vi "GetDataVersion.vi"(0 "session In":refnum<k35>, 5 "GEA2 Reference In":refnum<k24>, 11 "error In":errorcluster) -> (4 "session out":refnum<k35>, 8 "Data Version Out":cluster{"ERD Number":u16, "Data":string}[](array[cluster]), 15 "error out":errorcluster)   [LabVIEW 2023]
uses:
  D:/Common/LabVIEW GEA2 Toolkit/source/GEA3 DLL Source/GeaCommunication.dll
  Common/LabVIEW GEA2 Toolkit/source/GEA3 DLL Source/GeaCommunication.dll
  Common/LabVIEW GEA2 Toolkit/GEA3/type defs/Data Type.ctl
  Common/LabVIEW GEA2 Toolkit/GEA3/library/GEA2_Toolkit.lvlib
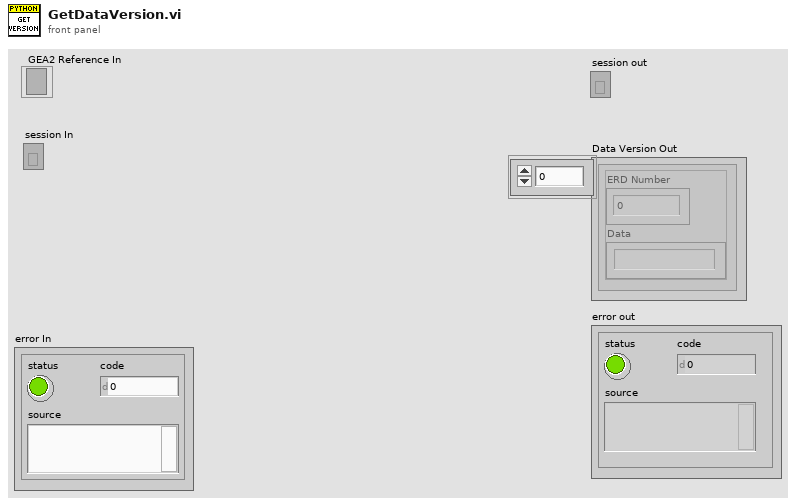
[diagram p1: front panel]
types:
  T1 = typedef "Data Type.ctl" = enum16{"string", "boolean", "uint8_t", "uint16_t", "uint32_t", "uint64_t", "int8_t", "int16_t", "int32_t", "int64_t"}
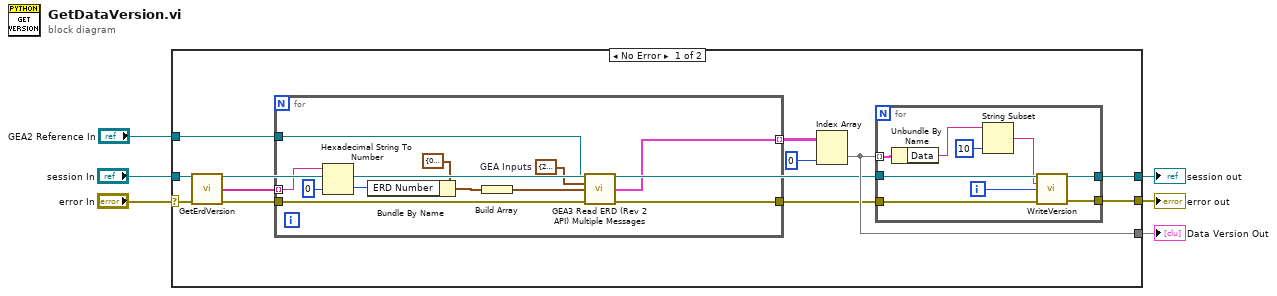
[diagram p0: block diagram]
diagram:
  n1 = case shown="No Error" "error In" {
    selector: "error In" -> [w8 w40]
    tunnel: [w15 _] -> w1
    tunnel: "GEA2 Reference In" -> [w11 _]
    tunnel: "session In" -> [w10 w39]
    tunnel: [w9 w39] -> w3
    tunnel: [w7 w40] -> w2
    frame No Error {
      n2 = call "GetErdVersion.vi"("session in"=w10, "error In"=w8) -> ("session Out"=w14:refnum<k35>, "Erds To Read"=w18:string[], "error Out"=w13:errorcluster)  [unwired: 11 in]
      n3 = for {
        tunnel: w11 -> [w38]
        tunnel: w13 -> [w37]
        tunnel: w18 -> [w32] mode=indexing
        tunnel: [w30] -> w17 mode=indexing
        tunnel: [w29] -> w12
        w36 = cluster{"Source":u8, "Destination":u8} {"Source"=229, "Destination"=192}  # GEA Inputs
        n4 = Hexadecimal String To Number(string=w32, default (0uL)=u16 0 ("ERD Number")) -> (number=w31:u16)  [unwired: 1 in, 1 out]
        n5 = Bundle By Name(cluster=cluster{"ERD Number":u16, "Data Type":T1} {"ERD Number"=0, "Data Type"=enum."string"} ("ERD Read Data In"), "ERD Number"=w31) -> (w35:cluster{"ERD Number":u16, "Data Type":T1})
        n6 = Build Array(w35) -> (w33:cluster{"ERD Number":u16, "Data Type":T1}[])
        n7 = call "GEA3 Read ERD (Rev 2 API) Multiple Messages.vi"("GEA2 Reference In"=w38, "GEA Inputs"=w36, "Read ERD List"=w33, "Error In"=w37) -> ("ERD Data Out"=w30:cluster{"ERD Number":u16, "Data":string}[], "Error Out"=w29:errorcluster)  [unwired: 8 in, 2 out]
      }
      n8 = Index Array(array=w17, index (col)=0 ("disabled index (col)")) -> (element=w15:cluster{"ERD Number":u16, "Data":string}[])  [unwired: 1 in]
      n9 = for {
        tunnel: w15 -> [w27] mode=indexing
        tunnel: w14 -> [w25]
        tunnel: [w26] -> w9
        tunnel: w12 -> [w24]
        tunnel: [w22] -> w7
        i -> [w23]
        n10 = Unbundle By Name(w27) -> ("Data"=w20:string)
        n11 = String Subset(string=w20, length (rest)=10 ("length (rest)")) -> (substring=w19:string)  [unwired: 1 in]
        n12 = call "WriteVersion.vi"("session in"=w25, "Data input"=w19, "index"=w23, "error In"=w24) -> ("session out"=w26:refnum<k35>, "error Out"=w22:errorcluster)  [unwired: 10 in]
      }
    }
    frame Error {
    }
  }
  "session out" <- w3
  "error out" <- w2
  "Data Version Out" <- w1
